vi "Temp2700Run.vi"(8 "error in":errorcluster, 10 "Run":bool, 11 "VISA resource name":refnum<visa-resource-name>) -> (0 "error out":errorcluster, 1 "Response (original)":string, 2 "Success":bool, 3 "VISA resource name out":refnum<visa-resource-name>)   [LabVIEW 2016]
uses:
  <instrlib>/Samwontech TEMP2xxx/Samwontech TEMP2xxx.lvlib
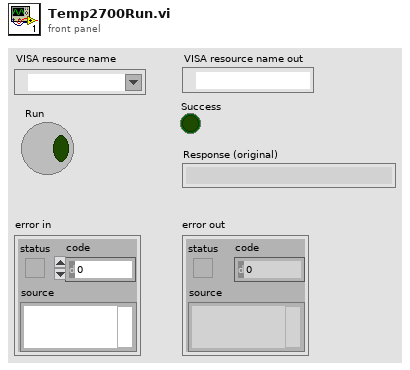
[diagram p1: front panel]
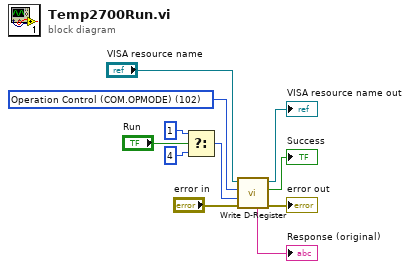
[diagram p0: block diagram]
diagram:
  w9 = u32 102 items=["Current PV (NPV)"=1, "Operation Control (COM.OPMODE)"=102, "Set Point on FIX operation (FIX.TSP)"=104, "Operation Mode (OP.MODE)"=106] ("D-Registers Map")
  n1 = Select(t=u32 1 ("Data"), s="Run", f=u32 4 ("Data")) -> (s? t:f=w2:u32)
  n2 = call <instrlib>:"Write D-Register.vi"("error in"="error in", "Data"=w2, "D-register number"=w9, "VISA resource name"="VISA resource name") -> ("error out"=→"error out":errorcluster, "Successfully"=→"Success":bool, "VISA resource name out"=→"VISA resource name out":refnum<visa-resource-name>, "Responce (original)"=→"Response (original)":string)  [unwired: 4 in]
